vi "tdms.waveform_to_csv.vi"(8 "error in":errorcluster, 10 "Formatted Channel Name":string, 11 "Waveform":waveform(dbl)) -> (0 "error out":errorcluster, 3 "new csv filepath":path)   [LabVIEW 2020, in "Nominal Client.lvclass"]
uses:
  Nominal Client.lvclass
  d82bedb3-8cc9-46d1-b6d5-f51039458690.vi
  <vilib>/LabVIEW Open Source Project/Epoch Date & Time/epoch.UNIX/Epoch.UNIX.lvclass
  C:/Program Files/National Instruments/LabVIEW 2020/vi.lib/LabVIEW Open Source Project/Epoch Date & Time/epoch/Epoch.lvclass
  <vilib>/LabVIEW Open Source Project/Epoch Date & Time/Get Epoch Time.vi
  <vilib>/Utility/file.llb/Write Delimited Spreadsheet (string).vi
  Nominal Client.lvclass/Nominal Client.ctl
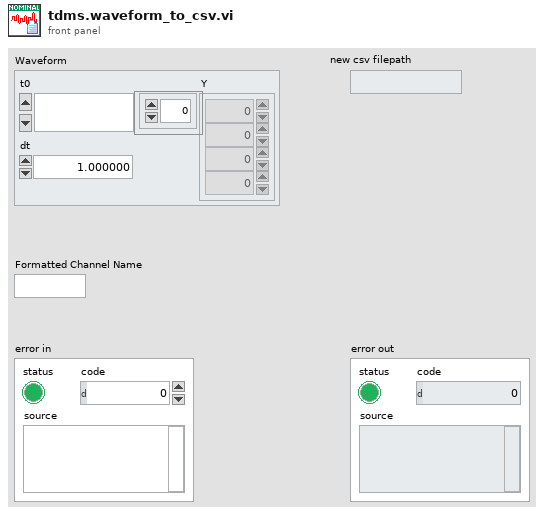
[diagram p1: front panel]
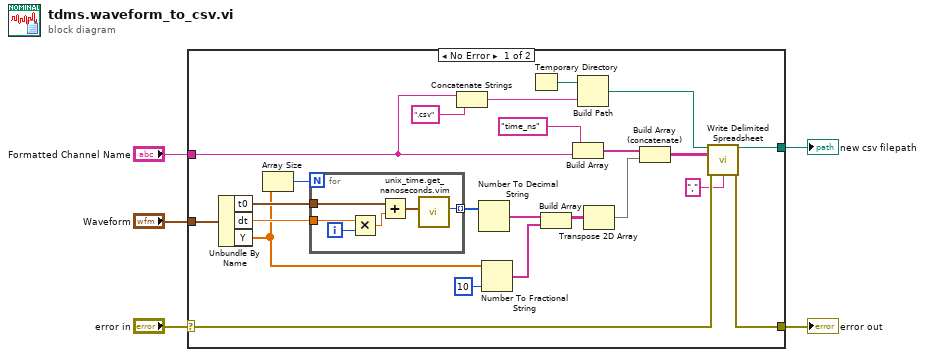
[diagram p0: block diagram]
diagram:
  n1 = case shown="No Error" "error in" {
    selector: "error in" -> [w7 w35]
    tunnel: "Formatted Channel Name" -> [w8 _]
    tunnel: [w15 w35] -> w3
    tunnel: [w14 _] -> w1
    tunnel: "Waveform" -> [w9 _]
    frame No Error {
      n2 = Unbundle By Name(w9) -> ("t0"=w28:timestamp, "dt"=w27:dbl, "Y"=w21:dbl[])
      n3 = Array Size(array=w21) -> (size(s)=w22:i32)
      n4 = for {
        N: w22 -> [_]
        tunnel: w28 -> [w32]
        tunnel: w27 -> [w33]
        tunnel: [w29] -> w25 mode=indexing
        i -> [w34]
        n5 = Multiply(x=w33, y=w34) -> (x*y=w31:dbl)
        n6 = Add(x=w32, y=w31) -> (x+y=w30:timestamp)
        n7 = call "unix_time.get_nanoseconds.vim"("Time Stamp (empty: now) [single or array]"=w30) -> ("UNIX time nanoseconds"=w29:i64)  [unwired: 10 in]
      }
      n8 = Concatenate Strings(w8, ".csv" ("string")) -> (w11:string)
      n9 = Number To Decimal String(number=w25) -> (decimal integer string=w24:string[])  [unwired: 1 in]
      n10 = Number To Fractional String(number=w21, precision (6)=i16 10) -> (F-format string=w20:string[])  [unwired: 2 in]
      n11 = Temporary Directory() -> (w13:path)
      n12 = Build Array(w24, w20) -> (w19:string[][])
      n13 = Build Array("time_ns", w8) -> (w23:string[])
      n14 = Build Path(base path=w13, name or relative path=w11) -> (appended path=w10:path)
      n15 = Transpose 2D Array(2D array=w19) -> (transposed array=w18:string[][])
      n16 = Build Array (concatenate)(w23, w18) -> (w16:string[][])
      n17 = call-poly <vilib>:"Write Delimited Spreadsheet.vi"("file path (dialog if empty)"=w10, "2D data"=w16, "error in (no error)"=w7, "delimiter (\\t)"="," ("delimiter (\\t)")) -> ("new file path (Not A Path if cancelled)"=w14:path, "error out"=w15:errorcluster)  [unwired: 10 in]
    }
    frame Error {
    }
  }
  "error out" <- w3
  "new csv filepath" <- w1
